vi "PH_BL-Master.check Start Phase over.vi"(0 "VI in":refnum<vi>, 5 "error in (no error)":errorcluster) -> (14 "VI out":refnum<vi>, 19 "error out":errorcluster)   [LabVIEW 2014, in "PH_BL-Master.lvlib"]
uses:
  PH_BL-Master.lvlib
panel:
  in  "Counter":i32
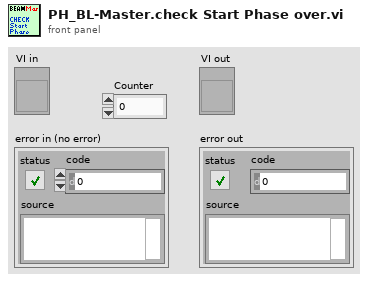
[diagram p1: front panel]
types:
  T1 = typedef "PH_BL-Master.lvlib/PH_BL-Master.i attribute.ctl" = cluster{"Remote controlled":bool, "Boolean Condition Service Subscriber":refnum<vi>[], "Picture Condition Service Subscriber":refnum<vi>[], "R2S":cluster{"GUI Ref":refnum<vi>, "State":bool}, "Vacua":cluster{"GUI Ref":refnum<vi>, "Limit":dbl, "Curr Value":dbl, "in range":bool}[], "O2 Inspection":cluster{"GUI Ref":refnum<vi>, "Concentration":dbl, "State":T2}[], "Boolean Status Service Subscriber":cluster{"GUI Ref":refnum<vi>, "Status":T2, "no Link?":bool, "Status Subscriber Class":T3}[], "Picture Status Service Subscriber":cluster{"GUI Ref":refnum<vi>, "Status":T2, "no Link?":bool, "Status Subscriber Class":T3}[], "6P 4Q Service Subscriber":cluster{"GUI Ref":refnum<vi>, "Selector":T4, "no Link?":bool}[], "Index of latest 6P 4Q changing Instance":i32, "Index of latest Picture Status changing Instance":i32, "Index of latest Boolean Status changing Instance":i32, "Vision ID on same Node":string, "Start Phase over?":bool, "GUI Ref Delete":refnum<vi>}
  T2 = typedef "PH_StatusHandler.lvlib/PH_StatusHandler.Status.ctl" = i16
  T3 = typedef "PH_BL-Master.lvlib/PH_BL-Master.Status Subscriber Class.ctl" = enum16{"unknown", "Switch", "BB", "6P Switch", "Switch GUI", "Switch and 6P State", "Force Sensor"}
  T4 = typedef "PH_4_Pos_Selector.lvlib/PH_4_Pos_Selector.Position Selector.ctl" = u16
  T5 = cluster{"GUI Ref":refnum<vi>, "Status":T2, "no Link?":bool, "Status Subscriber Class":T3}[]
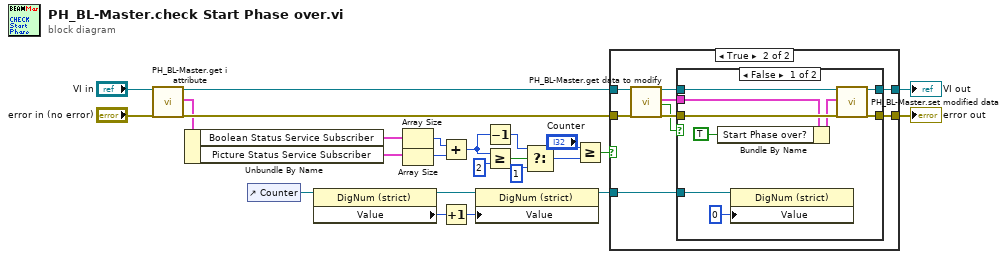
[diagram p0: block diagram]
diagram:
  n1 = call "PH_BL-Master.get i attribute.vi"("i ref in"="VI in", "error in (no error)"="error in (no error)") -> ("i ref out"=w11:refnum<vi>, "i attribute"=w23:T1, "error out"=w24:errorcluster)  [unwired: 15 in]
  n2 = Unbundle By Name(w23) -> ("Boolean Status Service Subscriber"=w20:T5, "Picture Status Service Subscriber"=w19:T5)
  n3 = control-ref of="Counter"() -> (w7:refnum<vi>)
  n4 = property class="DigNum (strict)"(reference=w7) -> (reference out=w6:refnum<vi>, "Value"=w5:i32)  [unwired: 1 in, 1 out]
  n5 = Array Size(array=w20) -> (size(s)=w18:i32)
  n6 = Array Size(array=w19) -> (size(s)=w17:i32)
  n7 = Add(x=w18, y=w17) -> (x+y=w13:i32)
  n8 = Increment(x=w5) -> (x+1=w4:i32)
  n9 = property class="DigNum (strict)"(reference=w6, "Value"=w4) -> (reference out=w1:refnum<vi>)  [unwired: 1 in, 1 out]
  n10 = Decrement(x=w13) -> (x-1=w15:i32)
  n11 = Greater Or Equal?(x=w13, y=2) -> (x >= y?=w14:bool)
  n12 = Select(t=w15, s=w14, f=1) -> (s? t:f=w3:i32)
  n13 = Greater Or Equal?(x="Counter", y=w3) -> (x >= y?=w8:bool)
  n14 = case shown="True" w8 {
    tunnel: w24 -> [w25 w35]
    tunnel: w11 -> [w26 w33]
    tunnel: [w25 w32] -> w10
    tunnel: [w26 w30] -> w9
    tunnel: w1 -> [_ w27]
    frame False {
    }
    frame True {
      n15 = call "PH_BL-Master.get data to modify.vi"("i ref in"=w33, "error in (no error)"=w35) -> ("i ref out"=w31:refnum<vi>, "i attribute"=w28:T1, "timed out"=w29:bool, "error out"=w34:errorcluster)  [unwired: 14 in]
      n16 = case shown="False" w29 {
        tunnel: w34 -> [w44 w45]
        tunnel: [w43 w45] -> w32
        tunnel: w31 -> [w42 w46]
        tunnel: [w41 w46] -> w30
        tunnel: w28 -> [w40 _]
        tunnel: w27 -> [w36 _]
        frame False {
          n17 = Bundle By Name(cluster=w40, "Start Phase over?"=TRUE) -> (w39:T1)
          n18 = property class="DigNum (strict)"(reference=w36, "Value"=0) -> ()  [unwired: 1 in, 2 out]
          n19 = call "PH_BL-Master.set modified data.vi"("i ref in"=w42, "i attribute"=w39, "error in (no error)"=w44) -> ("i ref out"=w41:refnum<vi>, "error out"=w43:errorcluster)  [unwired: 15 in]
        }
        frame True {
        }
      }
    }
  }
  "error out" <- w10
  "VI out" <- w9
